vi "OI_iPSM_Control_Remote.vi"() -> ()   [LabVIEW 2024]
panel:
  in  "SWITCH HEATER":bool
  in  "OK Button":bool
  in  "Magnet Controls":T1
  in  "Target Rate (A/min)":dbl format="%_5g"
  in  "Target Current (A)":dbl format="%_5g"
  in  "Ramp Controls":T2 {"Target Rate (T/min)" format="%_5g"; "Target Field (T)" format="%_5g"; "Target Rate (A/min)" format="%_5g"; "Target Current (A)" format="%_5g"}
  out "SW HTR CONFIRM":bool
  in  "Slew Rate":dbl=1.0 format="%#_4g"
  out "error out 3":errorcluster
  in  "Setpoint [T]":dbl format="%#_4g"
  in  "stop":bool
  in  "port":u16=3376
  in  "error in (no error) 2":errorcluster
  in  "Data mac ip address":string="mrl-dvh-elsa.mrl.illinois.edu"
  out "Field [T]":dbl=-17.9883723
  # "[T/min]"
  # "Note\n(1) Exception of the firewall should be configured.\n(2) With some (not all) connection with PC's, it is successful only when the VI is first executed. If the VI is stopped (normally or by aborting), \nthe subsequent connection is only possible with a new port number."
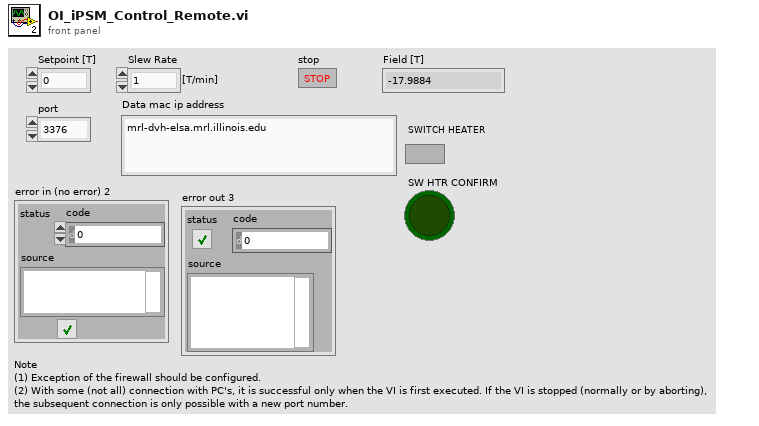
[diagram p1: front panel]
types:
  T1 = cluster{"CLAMP":bool, "HOLD":bool, "TO SET":bool, "TO ZERO":bool}
  T2 = cluster{"Target Current (A)":dbl, "Target Rate (A/min)":dbl, "Target Field (T)":dbl, "Target Rate (T/min)":dbl}
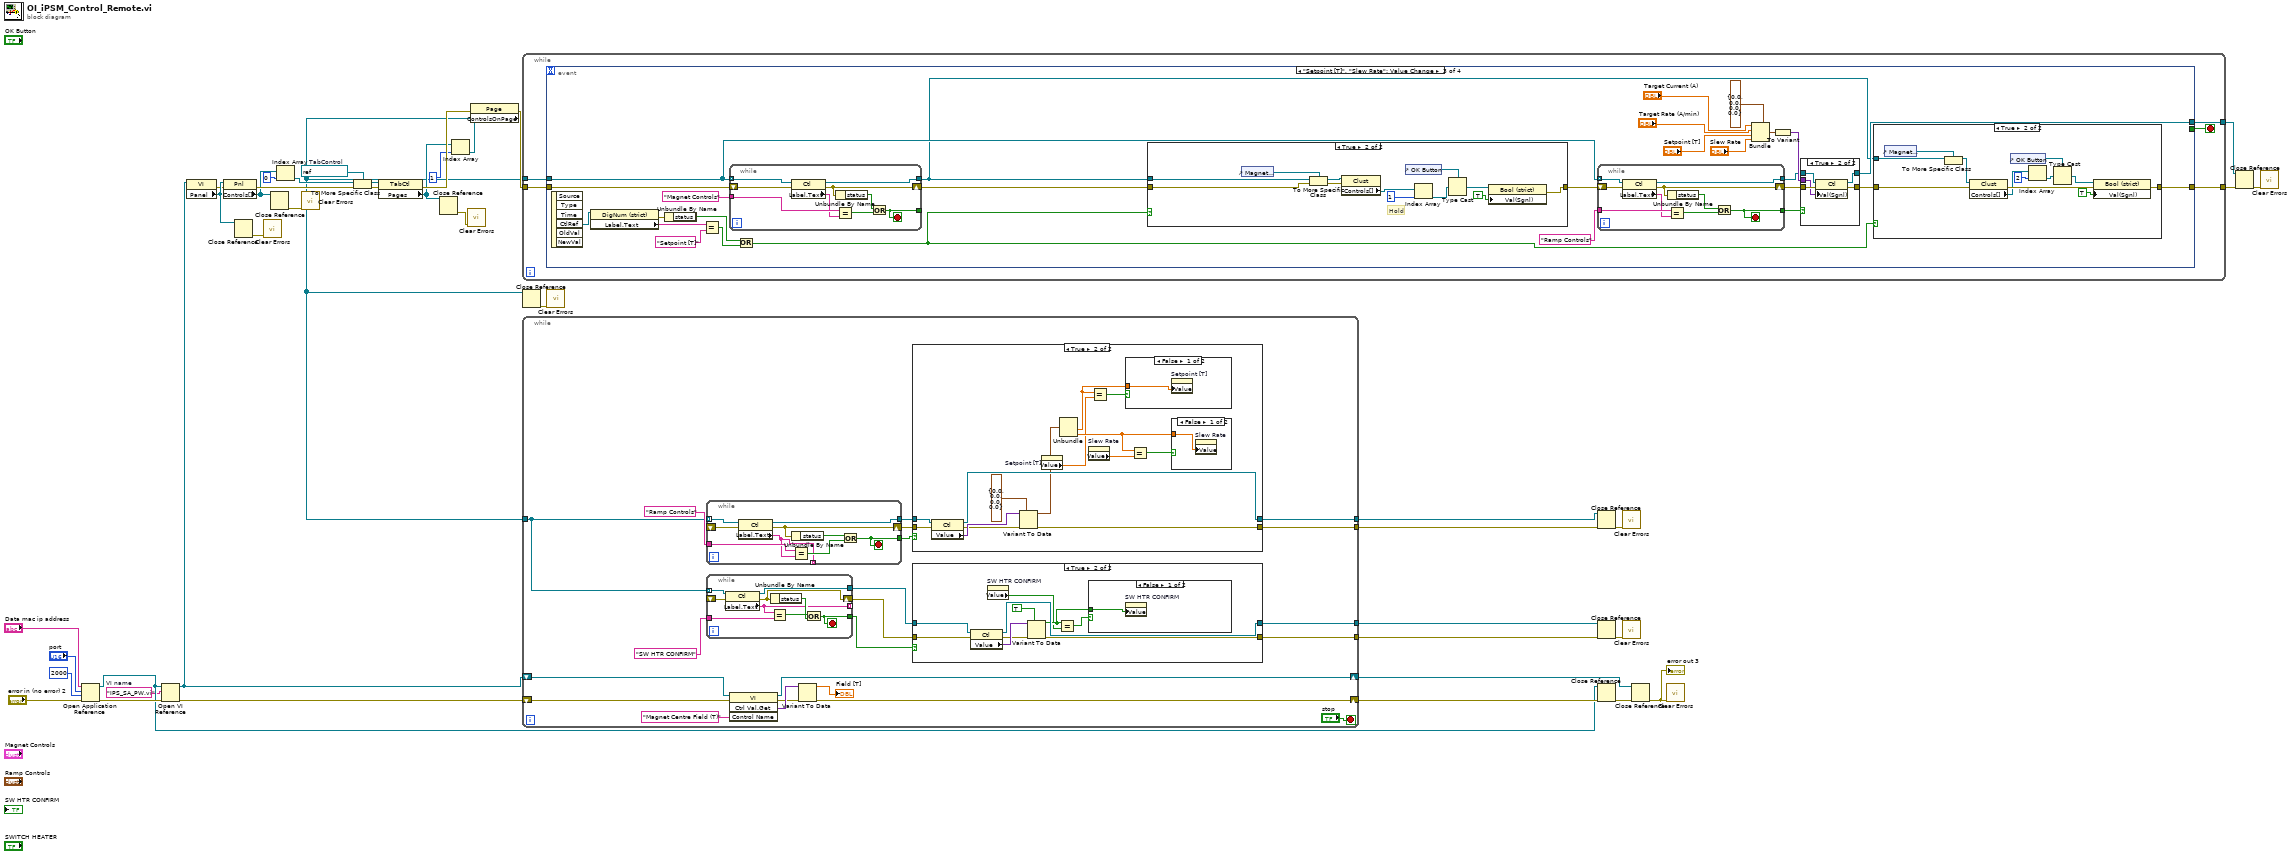
[diagram p0: block diagram]
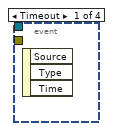
[diagram p2: hidden frame]
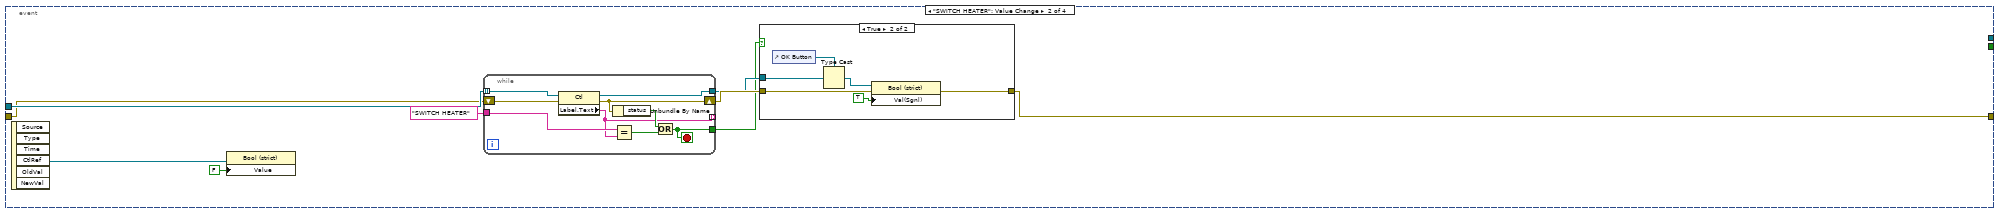
[diagram p3: hidden frame]
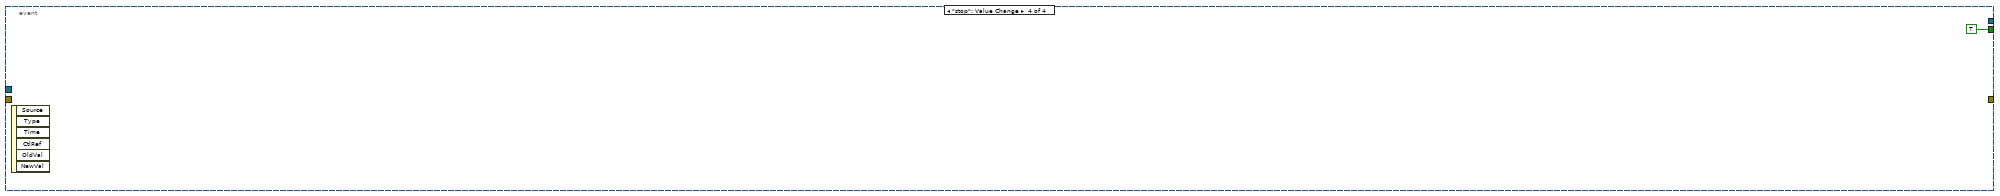
[diagram p8: hidden frame]
diagram:
  w14 = refnum<vi> refnum  # TabControl
  w33 = "IPS_SA_PW.vi"  # VI name
  n1 = Open Application Reference(8:"error in (no error) 2", 9:2000 ("timeout ms (60000)"), 10:"port", 11:"Data mac ip address") -> (0:w40:errorcluster, 3:w35:refnum<vi>)
  n2 = Open VI Reference(application reference (local)=w35, vi path=w33, error in (no error)=w40) -> (vi reference=w30:refnum<vi>, error out=w29:errorcluster)  [unwired: 3 in]
  n3 = property class="VI"(reference=w30) -> (error out=w17:errorcluster, "Panel"=w20:refnum<vi>)  [unwired: 1 in, 1 out]
  n4 = property class="Pnl"(reference=w20, error in=w17) -> (error out=w26:errorcluster, "Controls[]"=w22:refnum<vi>[])  [unwired: 1 out]
  n5 = Close Reference(reference=w20) -> (error out=w16:errorcluster)  [unwired: 1 in]
  n6 = call <vilib>:"Clear Errors.vi"("error in (no error)"=w16) -> ()  [unwired: 5 in, 2 out]
  n7 = Close Reference(reference=w22) -> (error out=w21:errorcluster)  [unwired: 1 in]
  n8 = Index Array(array=w22, index=0) -> (element=w18:refnum<vi>)
  n9 = call <vilib>:"Clear Errors.vi"("error in (no error)"=w21) -> ()  [unwired: 5 in, 2 out]
  n10 = To More Specific Class(target class=w14, reference=w18, error in=w26) -> (specific class reference=w19:refnum<vi>, error out=w27:errorcluster)
  n11 = property class="TabCtl"(reference=w19, error in=w27) -> (error out=w28:errorcluster, "Pages"=w24:refnum<vi>[])  [unwired: 1 out]
  n12 = Close Reference(reference=w24) -> (error out=w23:errorcluster)  [unwired: 1 in]
  n13 = Index Array(array=w24, index=1) -> (element=w25:refnum<vi>)
  n14 = call <vilib>:"Clear Errors.vi"("error in (no error)"=w23) -> ()  [unwired: 5 in, 2 out]
  n15 = property class="Page"(reference=w25, error in=w28) -> (error out=w12:errorcluster, "ControlsOnPage"=w5:refnum<vi>[])  [unwired: 1 out]
  n16 = while {
    tunnel: w12 -> [w45]
    tunnel: w5 -> [w44]
    tunnel: [w43] -> w7
    tunnel: [w42] -> w6
    stop <- w46 stop-if-true
    n17 = event shown="[2] \"Setpoint [T]\", \"Slew Rate\": Value Change" {
      selector: _ -> [_ _ _ _]
      dyn-events: _ -> [_ _ _ _]
      timeout: _ -> [_ _ _ _]
      tunnel: [_ _ _ TRUE] -> w46
      tunnel: [_ _ w73 _] -> w43
      tunnel: w45 -> [_ w54 w78 _]
      tunnel: w44 -> [_ w55 w79 _]
      tunnel: [_ w49 w77 _] -> w42
      event Timeout {
        n18 = event-data() -> ()  [unwired: 1 in, 3 out]
      }
      event "SWITCH HEATER": Value Change {
        n19 = event-data() -> ("CtlRef"=w48:refnum<vi>)  [unwired: 1 in, 5 out]
        n20 = property class="Bool (strict)"(reference=w48, "Value"=FALSE) -> ()  [unwired: 1 in, 2 out]
        n21 = while {
          tunnel: w55 -> [w71] mode=indexing
          tunnel: "SWITCH HEATER" ("Control Name") -> [w70]
          shift-right: [w67] -> w52
          shift-left: w54 -> [w69]
          tunnel: [w68] -> w51
          tunnel: [w64] -> w50
          tunnel: [w63] -> _ mode=indexing
          stop <- w64 stop-if-true
          n22 = property class="Ctl"(reference=w71, error in=w69) -> (reference out=w68:refnum<vi>, error out=w67:errorcluster, "Label.Text"=w63:string)
          n23 = Unbundle By Name(w67) -> ("status"=w66:bool)
          n24 = Equal?(x=w70, y=w63) -> (x = y?=w65:bool)
          n25 = Or(x=w66, y=w65) -> (x .or. y?=w64:bool)
        }
        n26 = case shown="True" w50 {
          tunnel: [w56 w62] -> w49
          tunnel: w52 -> [w56 w60]
          tunnel: w51 -> [_ w57]
          frame False {
          }
          frame True {
            n27 = control-ref of="OK Button"() -> (w61:refnum<vi>)
            n28 = Type Cast(type=w61, x=w57) -> (*(type *) &x=w59:refnum<vi>)
            n29 = property class="Bool (strict)"(reference=w59, error in=w60, "Val(Sgnl)"=TRUE ("Value (Signaling)")) -> (error out=w62:errorcluster)  [unwired: 1 out]
          }
        }
      }
      event "Setpoint [T]", "Slew Rate": Value Change {
        n30 = event-data() -> ("CtlRef"=w87:refnum<vi>)  [unwired: 1 in, 5 out]
        n31 = property class="DigNum (strict)"(reference=w87) -> (error out=w84:errorcluster, "Label.Text"=w86:string)  [unwired: 1 in, 1 out]
        n32 = Unbundle By Name(w84) -> ("status"=w83:bool)
        n33 = Equal?(x=w86, y="Setpoint [T]" ("Control Name")) -> (x = y?=w82:bool)
        n34 = while {
          tunnel: w79 -> [w120] mode=indexing
          tunnel: "Magnet Controls" ("Control Name") -> [w119]
          shift-right: [w116] -> w76
          shift-left: w78 -> [w118]
          tunnel: [w117] -> w72
          tunnel: [w113] -> _
          stop <- w113 stop-if-true
          n35 = property class="Ctl"(reference=w120, error in=w118) -> (reference out=w117:refnum<vi>, error out=w116:errorcluster, "Label.Text"=w112:string)
          n36 = Unbundle By Name(w116) -> ("status"=w115:bool)
          n37 = Equal?(x=w119, y=w112) -> (x = y?=w114:bool)
          n38 = Or(x=w115, y=w114) -> (x .or. y?=w113:bool)
        }
        n39 = Or(x=w83, y=w82) -> (x .or. y?=w75:bool)
        n40 = case shown="True" w75 {
          tunnel: w76 -> [w99 w108]
          tunnel: [w99 w107] -> w74
          tunnel: w72 -> [_ w100]
          frame False {
          }
          frame True {
            # "Hold"
            n41 = control-ref of="Magnet Controls"() -> (w110:refnum<vi>)
            n42 = To More Specific Class(target class=w110, reference=w100, error in=w108) -> (specific class reference=w101:refnum<vi>, error out=w109:errorcluster)
            n43 = property class="Clust"(reference=w101, error in=w109) -> ("Controls[]"=w102:refnum<vi>[])  [unwired: 2 out]
            n44 = control-ref of="OK Button"() -> (w105:refnum<vi>)
            n45 = Index Array(array=w102, index=1) -> (element=w106:refnum<vi>)
            n46 = Type Cast(type=w105, x=w106) -> (*(type *) &x=w104:refnum<vi>)
            n47 = property class="Bool (strict)"(reference=w104, "Val(Sgnl)"=TRUE) -> (error out=w107:errorcluster)  [unwired: 1 in, 1 out]
          }
        }
        n48 = while {
          tunnel: w79 -> [w149] mode=indexing
          tunnel: "Ramp Controls" ("Control Name") -> [w148]
          shift-right: [w145] -> w97
          shift-left: w74 -> [w147]
          tunnel: [w146] -> w94
          tunnel: [w142] -> w98
          stop <- w142 stop-if-true
          n49 = property class="Ctl"(reference=w149, error in=w147) -> (reference out=w146:refnum<vi>, error out=w145:errorcluster, "Label.Text"=w141:string)
          n50 = Unbundle By Name(w145) -> ("status"=w144:bool)
          n51 = Equal?(x=w148, y=w141) -> (x = y?=w143:bool)
          n52 = Or(x=w144, y=w143) -> (x .or. y?=w142:bool)
        }
        n53 = Bundle(cluster=T2 {"Target Current (A)"=0.0, "Target Rate (A/min)"=0.0, "Target Field (T)"=0.0, "Target Rate (T/min)"=0.0} ("Ramp Controls"), "Target Current (A)"="Target Current (A)", "Target Rate (A/min)"="Target Rate (A/min)", "Target Field (T)"="Setpoint [T]", "Target Rate (T/min)"="Slew Rate") -> (w91:T2)
        n54 = To Variant(anything=w91) -> (Variant=w95:variant)
        n55 = case shown="True" w98 {
          tunnel: w94 -> [w134 w139]
          tunnel: w97 -> [w135 w140]
          tunnel: [w135 w138] -> w81
          tunnel: [w134 w137] -> w73
          tunnel: w95 -> [_ w136]
          frame False {
          }
          frame True {
            n56 = property class="Ctl"(reference=w139, error in=w140, "Val(Sgnl)"=w136) -> (reference out=w137:refnum<vi>, error out=w138:errorcluster)
          }
        }
        n57 = case shown="True" w75 {
          tunnel: w81 -> [w121 w128]
          tunnel: [w121 w126] -> w77
          tunnel: w72 -> [_ w125]
          frame False {
          }
          frame True {
            n58 = control-ref of="Magnet Controls"() -> (w124:refnum<vi>)
            n59 = To More Specific Class(target class=w124, reference=w125) -> (specific class reference=w123:refnum<vi>)  [unwired: 1 in, 1 out]
            n60 = property class="Clust"(reference=w123, error in=w128) -> (error out=w127:errorcluster, "Controls[]"=w122:refnum<vi>[])  [unwired: 1 out]
            n61 = control-ref of="OK Button"() -> (w133:refnum<vi>)
            n62 = Index Array(array=w122, index=2) -> (element=w131:refnum<vi>)
            n63 = Type Cast(type=w133, x=w131) -> (*(type *) &x=w130:refnum<vi>)
            n64 = property class="Bool (strict)"(reference=w130, error in=w127, "Val(Sgnl)"=TRUE) -> (error out=w126:errorcluster)  [unwired: 1 out]
          }
        }
      }
      event "stop": Value Change {
        n65 = event-data() -> ()  [unwired: 1 in, 6 out]
      }
    }
  }
  n66 = Close Reference(reference=w5) -> (error out=w1:errorcluster)  [unwired: 1 in]
  n67 = while {
    shift-right: [w170] -> w34
    shift-left: w30 -> [w165]
    shift-right: [w172] -> w37
    shift-left: w29 -> [w164]
    tunnel: w5 -> [w161]
    tunnel: [w160] -> w10
    tunnel: [w159] -> w9
    tunnel: [w155] -> w3
    tunnel: [w154] -> w2
    stop <- "stop" stop-if-true
    n68 = while {
      tunnel: w161 -> [w194] mode=indexing
      tunnel: "Ramp Controls" ("Control Name") -> [w193]
      shift-right: [w190] -> w152
      shift-left: _ -> [w192]
      tunnel: [w191] -> w153
      tunnel: [w187] -> w151
      tunnel: [w186] -> _ mode=indexing
      stop <- w187 stop-if-true
      n69 = property class="Ctl"(reference=w194, error in=w192) -> (reference out=w191:refnum<vi>, error out=w190:errorcluster, "Label.Text"=w186:string)
      n70 = Unbundle By Name(w190) -> ("status"=w189:bool)
      n71 = Equal?(x=w193, y=w186) -> (x = y?=w188:bool)
      n72 = Or(x=w189, y=w188) -> (x .or. y?=w187:bool)
    }
    n73 = while {
      tunnel: w161 -> [w221] mode=indexing
      tunnel: "SW HTR CONFIRM" ("Control Name") -> [w220]
      shift-right: [w217] -> w157
      shift-left: _ -> [w219]
      tunnel: [w218] -> w158
      tunnel: [w214] -> w156
      tunnel: [w213] -> _ mode=indexing
      stop <- w214 stop-if-true
      n74 = property class="Ctl"(reference=w221, error in=w219) -> (reference out=w218:refnum<vi>, error out=w217:errorcluster, "Label.Text"=w213:string)
      n75 = Unbundle By Name(w217) -> ("status"=w216:bool)
      n76 = Equal?(x=w213, y=w220) -> (x = y?=w215:bool)
      n77 = Or(x=w216, y=w215) -> (x .or. y?=w214:bool)
    }
    n78 = invoke class="VI" method="Ctrl Val.Get"(reference=w165, error in=w164, "Control Name"="Magnet Centre Field (T)") -> (reference out=w170:refnum<vi>, error out=w168:errorcluster, "Get Control Value Variant"=w169:variant)  [unwired: 1 in, 1 out]
    n79 = Variant To Data(error in=w168, Variant=w169) -> (data=→"Field [T]":dbl, error out=w172:errorcluster)  [unwired: 1 in]
    n80 = case shown="True" w151 {
      tunnel: [w195 w208] -> w159
      tunnel: [w196 w209] -> w160
      tunnel: w153 -> [w196 w198]
      tunnel: w152 -> [w195 w197]
      frame False {
      }
      frame True {
        n81 = property class="Ctl"(reference=w198, error in=w197) -> (reference out=w209:refnum<vi>, error out=w207:errorcluster, "Value"=w210:variant)
        n82 = Variant To Data(error in=w207, type=T2 {"Target Current (A)"=0.0, "Target Rate (A/min)"=0.0, "Target Field (T)"=0.0, "Target Rate (T/min)"=0.0} ("Ramp Controls"), Variant=w210) -> (data=w203:T2, error out=w208:errorcluster)
        n83 = property on="Setpoint [T]" class="DigNum (strict)"() -> ("Value"=w200:dbl)  [unwired: 2 in, 2 out]
        n84 = Unbundle(w203) -> ("Target Field (T)"=w199:dbl, "Target Rate (T/min)"=w202:dbl)  [unwired: 2 out]
        n85 = property on="Slew Rate" class="DigNum (strict)"() -> ("Value"=w206:dbl)  [unwired: 2 in, 2 out]
        n86 = Equal?(x=w199, y=w200) -> (x = y?=w201:bool)
        n87 = case shown="False" w201 {
          tunnel: w199 -> [w211 _]
          frame False {
            n88 = property on="Setpoint [T]" class="DigNum (strict)"("Value"=w211) -> ()  [unwired: 2 in, 2 out]
          }
          frame True {
          }
        }
        n89 = Equal?(x=w202, y=w206) -> (x = y?=w205:bool)
        n90 = case shown="False" w205 {
          tunnel: w202 -> [w212 _]
          frame False {
            n91 = property on="Slew Rate" class="DigNum (strict)"("Value"=w212) -> ()  [unwired: 2 in, 2 out]
          }
          frame True {
          }
        }
      }
    }
    n92 = case shown="True" w156 {
      tunnel: w157 -> [w174 w184]
      tunnel: [w174 w181] -> w154
      tunnel: [w173 w182] -> w155
      tunnel: w158 -> [w173 w178]
      frame False {
      }
      frame True {
        n93 = property class="Ctl"(reference=w178, error in=w184) -> (reference out=w182:refnum<vi>, error out=w180:errorcluster, "Value"=w183:variant)
        n94 = property on="SW HTR CONFIRM" class="Bool (strict)"() -> ("Value"=w175:bool)  [unwired: 2 in, 2 out]
        n95 = Variant To Data(error in=w180, type=TRUE ("SW HTR CONFIRM"), Variant=w183) -> (data=w176:bool, error out=w181:errorcluster)
        n96 = Equal?(x=w176, y=w175) -> (x = y?=w179:bool)
        n97 = case shown="False" w179 {
          tunnel: w176 -> [w185 _]
          frame False {
            n98 = property on="SW HTR CONFIRM" class="Bool (strict)"("Value"=w185) -> ()  [unwired: 2 in, 2 out]
          }
          frame True {
          }
        }
      }
    }
  }
  n99 = call <vilib>:"Clear Errors.vi"("error in (no error)"=w1) -> ()  [unwired: 5 in, 2 out]
  n100 = Close Reference(reference=w10, error in (no error)=w9) -> (error out=w11:errorcluster)
  n101 = Close Reference(reference=w3, error in (no error)=w2) -> (error out=w4:errorcluster)
  n102 = Close Reference(reference=w35, error in (no error)=w37) -> (error out=w36:errorcluster)
  n103 = call <vilib>:"Clear Errors.vi"("error in (no error)"=w11) -> ()  [unwired: 5 in, 2 out]
  n104 = call <vilib>:"Clear Errors.vi"("error in (no error)"=w4) -> ()  [unwired: 5 in, 2 out]
  n105 = Close Reference(reference=w34, error in (no error)=w36) -> (error out=w31:errorcluster)
  "error out 3" <- w31
  n106 = call <vilib>:"Clear Errors.vi"("error in (no error)"=w31) -> ()  [unwired: 5 in, 2 out]
  n107 = Close Reference(reference=w7, error in (no error)=w6) -> (error out=w8:errorcluster)
  n108 = call <vilib>:"Clear Errors.vi"("error in (no error)"=w8) -> ()  [unwired: 5 in, 2 out]
